vi "implementation_setpoint.vi"(2 "Meas":T2 {"Ud" format="%#.2f"; "P" format="%#.2f"; "Q" format="%#.2f"}, 3 "param":T1={"Srated"=25000.0, "eta [pu]"=0.98, "model"={"in-states"={"v1"=0.0, "v2"=0.0, "SoC"=0.0}, "output"={"V"=0.0, "Zeq"=0.0, "Eeq"=0.0}}} {"model"."output"."Eeq" format="%#.6g"; "model"."output"."Zeq" format="%#.6g"; "eta [pu]" format="%#_13g"}, 4 "PacLims (in)":cluster{"Pmax":dbl, "Pmin":dbl}, 5 "REQ":T3) -> (0 "send_cmd?":bool, 1 "uc":cluster{"Pc":dbl, "Qc":dbl})   [LabVIEW 2021]
doc: "This VI computes the projected values of the request setpoint. It takes as inputs the active and reactive power boundaries (Ptmin, Ptmax, Srmax) and the request setpoint (Preq, Qreq). It returns as outputs the projected values of the request setpoint inside the active and reactive power boundaries (P'bt, Q'bt), and a graph in the PQ plane showing the position of the request setpoint and of the projected one. \n\nIt is based on a simple gradient projection method. If the request setpoint lies inside the active and reactive power boundaries, the projected value correspond to the request setpoint. If the request active power lies inside the active power boundaries, the projected value will assume the value of the request, if it does not, the projected value will assume the value of Ptmin or Ptmax. The corresponding phasor is computed. If the magnitude of the phasor is lower or equal than the maximum complex power Srmax, the magnitude of the projected value will assume the value of the request, if it is not the magnitude of the projected value will assume the value of Srmax."
uses:
  General purpose/REQ.ctl
  General purpose/MEAS.ctl
  General purpose/agent-variables.ctl
panel:
  in  "errorQ":bool
  in  "errorP":bool
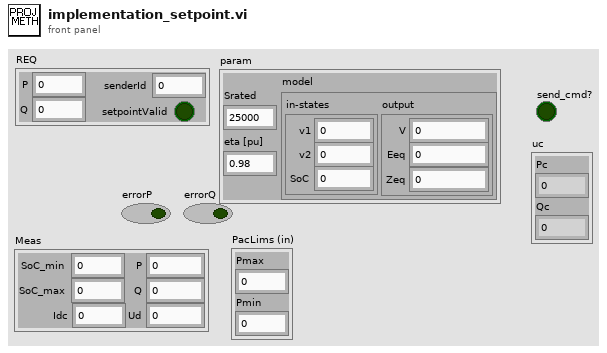
[diagram p1: front panel]
types:
  T1 = typedef "agent-variables.ctl" = cluster{"Srated":dbl, "eta [pu]":dbl, "model":cluster{"in-states":cluster{"v1":dbl, "v2":dbl, "SoC":dbl}, "output":cluster{"V":dbl, "Zeq":dbl, "Eeq":dbl}}}
  T2 = typedef "MEAS.ctl" = cluster{"P":dbl, "Q":dbl, "SoC_max":dbl, "SoC_min":dbl, "Ud":dbl, "Idc":dbl}
  T3 = typedef "REQ.ctl" = cluster{"P":dbl, "Q":dbl, "senderId":u32, "setpointValid":bool}
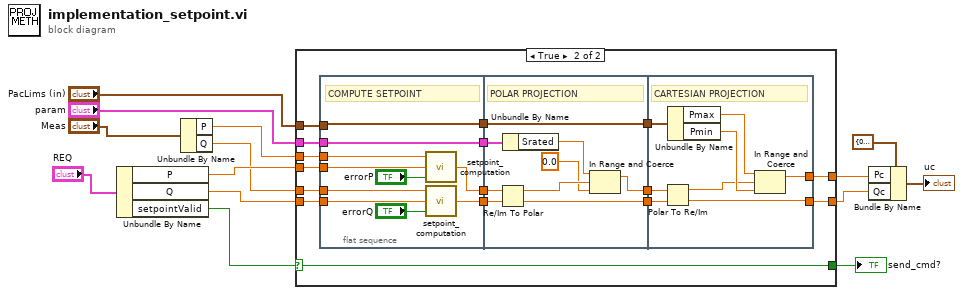
[diagram p0: block diagram]
diagram:
  n1 = Unbundle By Name("REQ") -> ("P"=w12:dbl, "Q"=w13:dbl, "setpointValid"=w9:bool)
  n2 = Unbundle By Name("Meas") -> ("P"=w11:dbl, "Q"=w10:dbl)
  n3 = case shown="True" w9 {
    selector: w9 -> [w15 w23]
    tunnel: [w17 w29] -> w6
    tunnel: [w16 w28] -> w1
    tunnel: w11 -> [w17 w27]
    tunnel: w12 -> [_ w26]
    tunnel: w10 -> [w16 w25]
    tunnel: w13 -> [_ w24]
    tunnel: [w15 w23] -> w14
    tunnel: "param" -> [_ w21]
    tunnel: "PacLims (in)" -> [_ w18]
    frame False {
    }
    frame True {
      n4 = flat-sequence {
        tunnel: [w43] -> w33
        tunnel: [w37] -> w32
        tunnel: w27 -> [w42]
        tunnel: w26 -> [w41]
        tunnel: w25 -> [w36]
        tunnel: w24 -> [w35]
        tunnel: w21 -> [w39]
        tunnel: [w39] -> w22
        tunnel: w18 -> [w38]
        tunnel: [w38] -> w20
        tunnel: [w47] -> w31
        tunnel: [w46] -> w30
        tunnel: w33 -> [w50]
        tunnel: w32 -> [w49]
        tunnel: w22 -> [w45]
        tunnel: w20 -> [w44]
        tunnel: [w44] -> w19
        tunnel: w31 -> [w56]
        tunnel: [w53] -> w28
        tunnel: w30 -> [w55]
        tunnel: [w58] -> w29
        tunnel: w19 -> [w57]
        frame #0 {
          # "COMPUTE SETPOINT"
          n5 = call "setpoint_computation.vi"("activate"="errorP", "Req"=w41, "Meas"=w42) -> ("SP"=w43:dbl)
          n6 = call "setpoint_computation.vi"("activate"="errorQ", "Req"=w35, "Meas"=w36) -> ("SP"=w37:dbl)
        }
        frame #1 {
          # "POLAR PROJECTION"
          n7 = Re/Im To Polar(2:w49, 3:w50) -> (0:w46:dbl, 1:w52:dbl)
          n8 = Unbundle By Name(w45) -> ("Srated"=w48:dbl)
          n9 = In Range and Coerce(upper limit=w48, x=w52, lower limit=0.0) -> (coerced(x)=w47:dbl)  [unwired: 1 out]
        }
        frame #2 {
          # "CARTESIAN PROJECTION"
          n10 = Polar To Re/Im(2:w55, 3:w56) -> (0:w53:dbl, 1:w54:dbl)
          n11 = Unbundle By Name(w57) -> ("Pmax"=w60:dbl, "Pmin"=w59:dbl)
          n12 = In Range and Coerce(upper limit=w60, x=w54, lower limit=w59) -> (coerced(x)=w58:dbl)  [unwired: 1 out]
        }
      }
    }
  }
  "send_cmd?" <- w14
  n13 = Bundle By Name(cluster=cluster{"Pc":dbl, "Qc":dbl} {"Pc"=0.0, "Qc"=0.0} ("uc"), "Pc"=w6, "Qc"=w1) -> (→"uc":cluster{"Pc":dbl, "Qc":dbl})
